vi "Main.vi"() -> ()   [LabVIEW 2010]
panel:
  out "Counter2":dbl
  out "Counter1":dbl
  in  "stop":bool
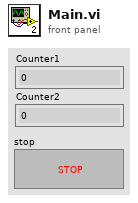
[diagram p1: front panel]
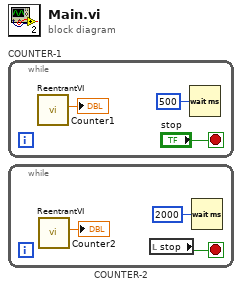
[diagram p0: block diagram]
diagram:
  n1 = while "COUNTER-1" {
    stop <- "stop" stop-if-true
    n2 = call "ReentrantVI.vi"() -> ("Counter"=→"Counter1":dbl)  [unwired: 11 in]
    n3 = Wait (ms)(milliseconds to wait=u32 500) -> ()  [unwired: 1 out]
  }
  n4 = while "COUNTER-2" {
    stop <- w6 stop-if-true
    n5 = call "ReentrantVI.vi"() -> ("Counter"=→"Counter2":dbl)  [unwired: 11 in]
    n6 = local read "stop"() -> (w6:bool)
    n7 = Wait (ms)(milliseconds to wait=u32 2000) -> ()  [unwired: 1 out]
  }
